vi "AVS_GetList.vi"(0 "ListSizeInput":u32, 7 "RequiredSizeInput":u32, 11 "ListInpit":u8[](array[numeric])) -> (4 "ListSizeOutput":u32, 8 "RequiredSizeOutput":u32, 15 "List Output":u8[](array[numeric]))   [LabVIEW 2013, in "Avantes Spectrometer Functions.lvlib"]
uses:
  Avantes Spectrometer Functions.lvlib
  AvantesSpectrometer2/polling_mc/AS5216.dll
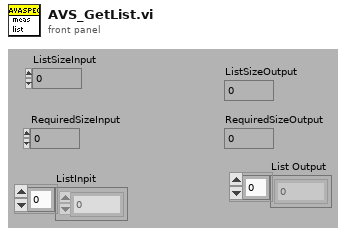
[diagram p1: front panel]
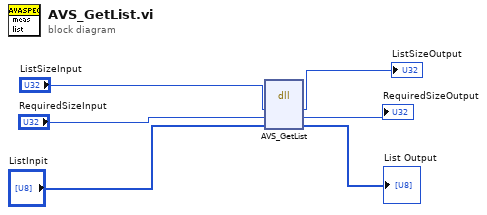
[diagram p0: block diagram]
diagram:
  n1 = dll-call lib="C:/Users/dhstuart/Dropbox/CLTC/AvantesSpectrometer2/polling_mc/AS5216.dll" fn="AVS_GetList"("a_ListSize"="ListSizeInput", "a_pRequiredSize"="RequiredSizeInput", "a_pList"="ListInpit") -> ("a_ListSize"=→"ListSizeOutput":u32, "a_pRequiredSize"=→"RequiredSizeOutput":u32, "a_pList"=→"List Output":u8[])  [unwired: 4 in, 2 out]
